vi "_Copy 1.vi"(0 "XRef":T5, 1 "State In":T1) -> (14 "Reply":T3, 15 "Fatal Error Out":T2, 16 "State Out":T1)   [LabVIEW 2014, in "JKISM++ DebugTool.xnode"]
uses:
  JKISM++ DebugTool.xnode
  <vilib>/XNodeSupport/XNodeXNodeRef.ctl
  _State 1.ctl
  <vilib>/XNodeSupport/XNodeStringArray.ctl
  <vilib>/XNodeSupport/XNodeString.ctl
  <vilib>/XNodeSupport/XNodeErrorCluster.ctl
  <vilib>/XNodeSupport/NI_XNodeSupport.lvlib
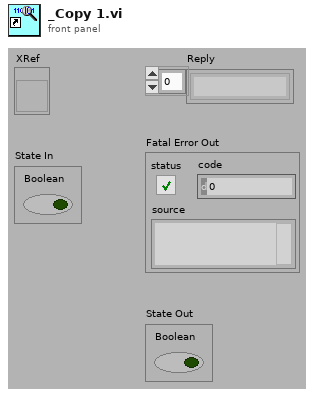
[diagram p1: front panel]
types:
  T1 = typedef "JKISM++ DebugTool.xnode/_State 1.ctl" = cluster{"Boolean":bool}
  T2 = typedef "NI_XNodeSupport.lvlib/XNodeErrorCluster.ctl" = errorcluster
  T3 = typedef "NI_XNodeSupport.lvlib/XNodeStringArray.ctl" = T4[]
  T4 = typedef "NI_XNodeSupport.lvlib/XNodeString.ctl" = string
  T5 = typedef "NI_XNodeSupport.lvlib/XNodeXNodeRef.ctl" = refnum<vi>
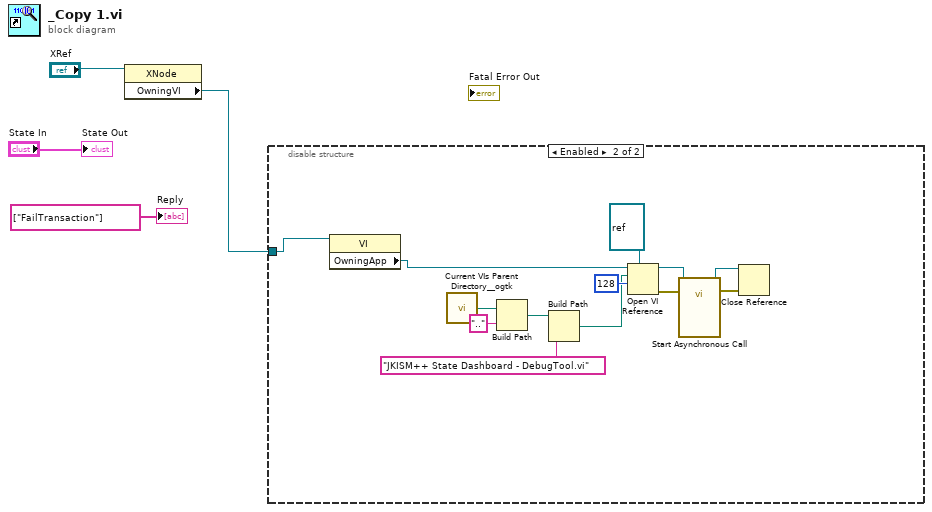
[diagram p0: block diagram]
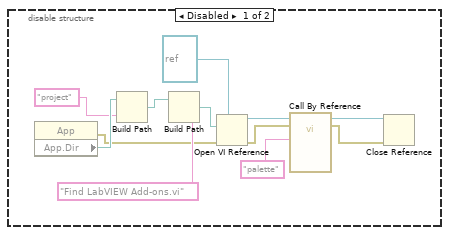
[diagram p2: hidden frame]
diagram:
  n1 = property class="XNode"(reference="XRef") -> ("OwningVI"=w1:refnum<vi>)  [unwired: 1 in, 2 out]
  n2 = disable-structure shown="Enabled" {
    disable-tunnel: w1 -> [_ w18]
    frame Disabled {
      n3 = property class="App"() -> (error out=w11:errorcluster, "App.Dir"=w16:path)  [unwired: 2 in, 1 out]
      n4 = Build Path(base path=w16, name or relative path="project") -> (appended path=w14:path)
      n5 = Build Path(base path=w14, name or relative path="Find LabVIEW Add-ons.vi") -> (appended path=w12:path)
      n6 = Open VI Reference(type specifier VI Refnum (for type only)=refnum<vi> refnum ("reference"), vi path=w12, error in (no error)=w11) -> (vi reference=w9:refnum<vi>, error out=w6:errorcluster)  [unwired: 3 in]
      n7 = call-by-ref "?"(reference=w9, error in=w6, "Source"="palette") -> (reference out=w5:refnum<vi>, error out=w7:errorcluster)  [unwired: 11 in]
      n8 = Close Reference(reference=w5, error in (no error)=w7) -> ()  [unwired: 1 out]
    }
    frame Enabled {
      n9 = property class="VI"(reference=w18) -> ("OwningApp"=w17:refnum<vi>)  [unwired: 1 in, 2 out]
      n10 = call <userlib>:"Current VIs Parent Directory__ogtk.vi"() -> ("Parent Directory (+ Relative)"=w29:path)  [unwired: 5 in]
      n11 = Build Path(base path=w29, name or relative path="..") -> (appended path=w27:path)
      n12 = Build Path(base path=w27, name or relative path="JKISM++ State Dashboard - DebugTool.vi") -> (appended path=w20:path)
      n13 = Open VI Reference(type specifier VI Refnum (for type only)=refnum<vi> refnum, application reference (local)=w17, vi path=w20, options=128) -> (vi reference=w22:refnum<vi>, error out=w21:errorcluster)  [unwired: 2 in]
      n14 = call-by-ref "Start Asynchronous Call"(reference=w22, error in=w21) -> (reference out=w24:refnum<vi>, error out=w23:errorcluster)  [unwired: 12 in]
      n15 = Close Reference(reference=w24, error in (no error)=w23) -> ()  [unwired: 1 out]
    }
  }
  "Reply" <- T3 ["FailTransaction"] ("Reply")
  "State Out" <- "State In"
